vi "USB_DAQ__EEPROM_Test_Array_WRITE_24C32.vi"() -> ()   [LabVIEW 2022 SP3]
panel:
  in  "Tx.Array":u8[](array[numeric])=[1, 2, 3, 4, 5, 6, 7, 8] format="%02x"
  in  "stop":bool
  out "Page.ACK0":bool
  in  "Page.Address0":u8 format="%02x"
  out "All.Acks.OK":bool
  in  "Page.Address1":u8 format="%02x"
  out "Page.ACK1":bool
  out "Addr.ACK":bool
  in  "24C32.Address":u8=87 format="%02x"
  in  "Write":bool
  # "EEPROM 24C32 ARRAY WRITE"
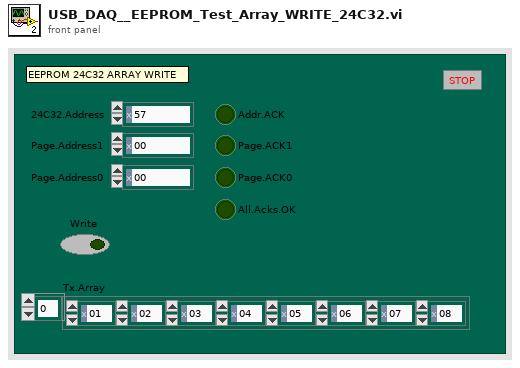
[diagram p1: front panel]
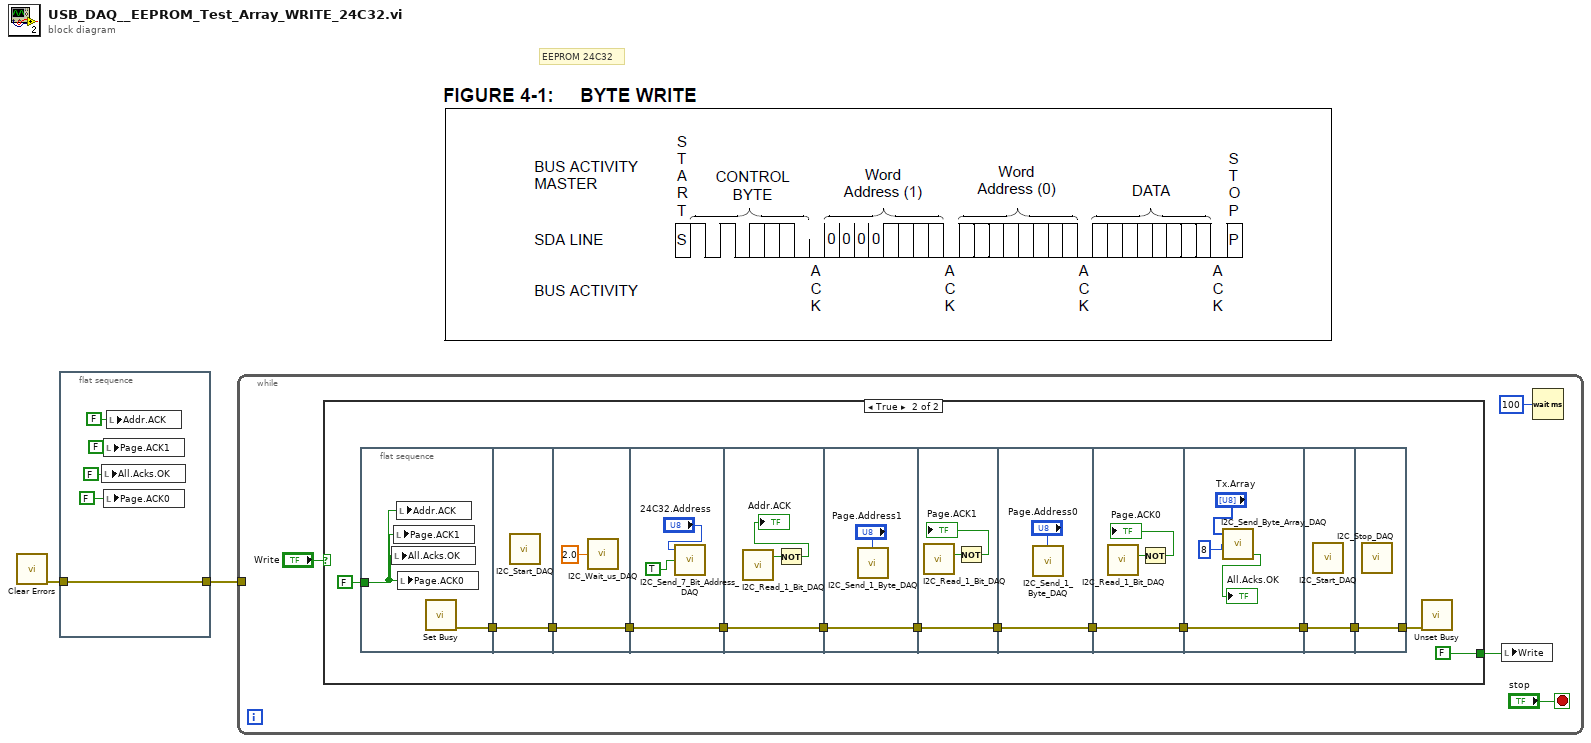
[diagram p0: block diagram]
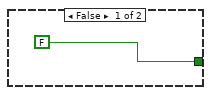
[diagram p2: hidden frame]
diagram:
  # "EEPROM 24C32"
  n1 = call <vilib>:"Clear Errors.vi"() -> ("error out"=w1:errorcluster)  [unwired: 6 in, 1 out]
  n2 = flat-sequence {
    tunnel: w1 -> [w7]
    tunnel: [w7] -> w2
    frame #0 {
      n3 = local write "All.Acks.OK"(FALSE ("Data.ACK")) -> ()
      n4 = local write "Page.ACK1"(FALSE ("TX.ACK")) -> ()
      n5 = local write "Page.ACK0"(FALSE ("Page.ACK0")) -> ()
      n6 = local write "Addr.ACK"(FALSE ("ACK_OK")) -> ()
    }
  }
  n7 = while {
    tunnel: w2 -> [_]
    stop <- "stop" stop-if-true
    n8 = case shown="True" "Write" {
      tunnel: [FALSE ("Test") FALSE ("Test")] -> w9
      frame False {
      }
      frame True {
        n9 = flat-sequence {
          tunnel: FALSE ("Data.ACK") -> [w28]
          tunnel: [w27] -> w14
          tunnel: [w29] -> w15
          tunnel: w14 -> [w29]
          tunnel: [w30] -> w16
          tunnel: w15 -> [w30]
          tunnel: [w32] -> w17
          tunnel: w16 -> [w32]
          tunnel: [w35] -> w18
          tunnel: w17 -> [w35]
          tunnel: [w38] -> w19
          tunnel: w18 -> [w38]
          tunnel: [w40] -> w20
          tunnel: w19 -> [w40]
          tunnel: [w43] -> w21
          tunnel: w20 -> [w43]
          tunnel: [w45] -> w22
          tunnel: w21 -> [w45]
          tunnel: [w48] -> w23
          tunnel: w22 -> [w48]
          tunnel: [w52] -> w24
          tunnel: w23 -> [w52]
          tunnel: [w53] -> w13
          tunnel: w24 -> [w53]
          frame #0 {
            n10 = local write "All.Acks.OK"(w28) -> ()
            n11 = local write "Page.ACK1"(w28) -> ()
            n12 = local write "Addr.ACK"(w28) -> ()
            n13 = local write "Page.ACK0"(w28) -> ()
            n14 = call <vilib>:"Set Busy.vi"() -> ("error out"=w27:errorcluster)  [unwired: 10 in, 1 out]
          }
          frame #1 {
            n15 = call "I2C_Start_DAQ.vi"() -> ()  [unwired: 6 in]
          }
          frame #2 {
            n16 = call "I2C_Wait_us_DAQ.vi"("Factor"=2.0) -> ()  [unwired: 5 in]
          }
          frame #3 {
            n17 = call "I2C_Send_7_Bit_Address_DAQ.vi"("Write or Read?"=TRUE, "Receiver_7_Bit_Address"="24C32.Address") -> ()  [unwired: 1 in]
          }
          frame #4 {
            n18 = call "I2C_Read_1_Bit_DAQ.vi"() -> ("RX_Bit_Out"=w37:bool)  [unwired: 2 in]
            n19 = Not(x=w37) -> (.not. x?=→"Addr.ACK":bool)
          }
          frame #5 {
            n20 = call "I2C_Send_1_Byte_DAQ.vi"("Byte_To_Send"="Page.Address1") -> ()  [unwired: 2 in]
          }
          frame #6 {
            n21 = call "I2C_Read_1_Bit_DAQ.vi"() -> ("RX_Bit_Out"=w42:bool)  [unwired: 2 in]
            n22 = Not(x=w42) -> (.not. x?=→"Page.ACK1":bool)
          }
          frame #7 {
            n23 = call "I2C_Send_1_Byte_DAQ.vi"("Byte_To_Send"="Page.Address0") -> ()  [unwired: 2 in]
          }
          frame #8 {
            n24 = call "I2C_Read_1_Bit_DAQ.vi"() -> ("RX_Bit_Out"=w47:bool)  [unwired: 2 in]
            n25 = Not(x=w47) -> (.not. x?=→"Page.ACK0":bool)
          }
          frame #9 {
            n26 = call "I2C_Send_Byte_Array_DAQ.vi"("Tx.Byte.Count"=8, "Tx.Array"="Tx.Array") -> ("ALL.ACKS.OK"=→"All.Acks.OK":bool)
          }
          frame #10 {
            n27 = call "I2C_Start_DAQ.vi"() -> ()  [unwired: 6 in]
          }
          frame #11 {
            n28 = call "I2C_Stop_DAQ.vi"() -> ()  [unwired: 6 in]
          }
        }
        n29 = call <vilib>:"Unset Busy.vi"("error in (no error)"=w13) -> ()  [unwired: 10 in, 1 out]
      }
    }
    n30 = local write "Write"(w9) -> ()
    n31 = Wait (ms)(milliseconds to wait=u32 100) -> ()  [unwired: 1 out]
  }
